vi "Estrai MW Contigui.vi"(10 "MW LETTURE":T1(array[cluster])) -> (1 "Number MW":i32[](array[numeric]), 2 "ArrayMW":i32[](array[numeric]))   [LabVIEW 2019]
panel:
  out "x = y?":bool
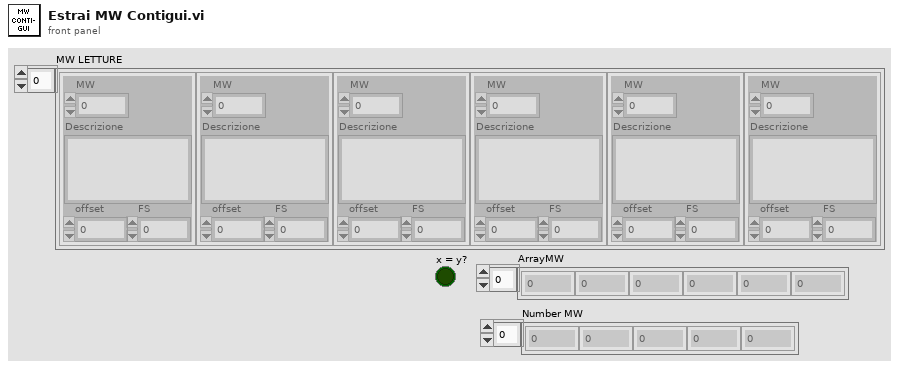
[diagram p1: front panel]
types:
  T1 = cluster{"MW":dbl, "Descrizione":string, "offset":dbl, "FS":dbl}[]
  T2 = cluster{"MW":dbl, "Descrizione":string, "offset":dbl, "FS":dbl}
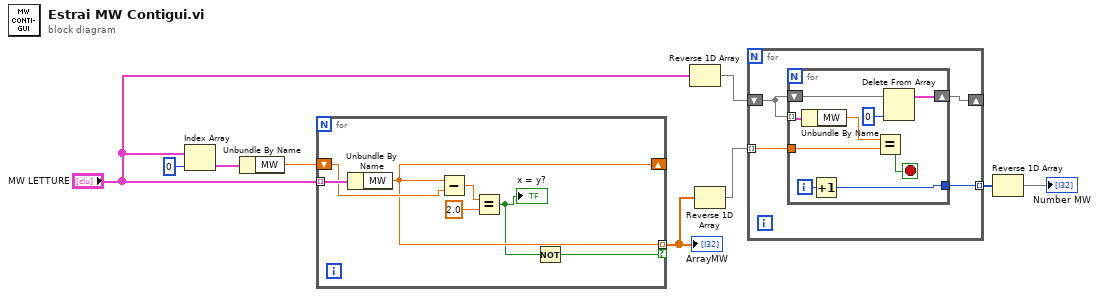
[diagram p0: block diagram]
diagram:
  n1 = Index Array(array="MW LETTURE", index=0) -> (element=w8:T2)
  n2 = Unbundle By Name(w8) -> ("MW"=w7:dbl)
  n3 = for {
    tunnel: "MW LETTURE" -> [w16] mode=indexing
    shift-right: [w12] -> _
    shift-left: w7 -> [w15]
    tunnel: [w12] -> w6 mode=indexing if=w11
    n4 = Unbundle By Name(w16) -> ("MW"=w12:dbl)
    n5 = Subtract(x=w12, y=w15) -> (x-y=w14:dbl)
    n6 = Equal?(x=w14, y=2.0) -> (x = y?=w10:bool)
    "x = y?" <- w10
    n7 = Not(x=w10) -> (.not. x?=w11:bool)
  }
  "ArrayMW" <- w6
  n8 = Reverse 1D Array(array="MW LETTURE") -> (reversed array=w3:T1)
  n9 = Reverse 1D Array(array=w6) -> (reversed array=w5:dbl[])
  n10 = for {
    tunnel: w5 -> [w20] mode=indexing
    shift-right: [w18] -> _
    shift-left: w3 -> [w19]
    tunnel: [w17] -> w2 mode=indexing
    n11 = for {
      tunnel: w19 -> [w29] mode=indexing
      tunnel: w20 -> [w27]
      shift-right: [w23] -> w18
      shift-left: w19 -> [w25]
      tunnel: [w21] -> w17
      i -> [w22]
      stop <- w26 stop-if-true
      n12 = Unbundle By Name(w29) -> ("MW"=w28:dbl)
      n13 = Increment(x=w22) -> (x+1=w21:i32)
      n14 = Equal?(x=w28, y=w27) -> (x = y?=w26:bool)
      n15 = Delete From Array(array=w25, index=0) -> (array with subset deleted=w23:T1)  [unwired: 1 in, 1 out]
    }
  }
  n16 = Reverse 1D Array(array=w2) -> (reversed array=→"Number MW":i32[])
